vi "Create file path.vi"(11 "# photos":i32) -> (3 "Path OUT":path)   [LabVIEW 2018]
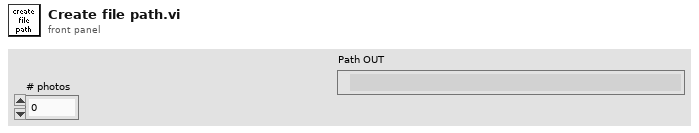
[diagram p1: front panel]
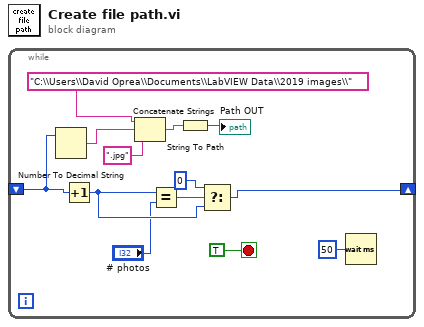
[diagram p0: block diagram]
diagram:
  n1 = while {
    shift-right: [w9] -> _
    shift-left: _ -> [w1]
    stop <- TRUE stop-if-true
    n2 = Number To Decimal String(number=w1) -> (decimal integer string=w8:string)  [unwired: 1 in]
    n3 = Increment(x=w1) -> (x+1=w10:i32)
    n4 = Concatenate Strings("C:\\Users\\David Oprea\\Documents\\LabVIEW Data\\2019 images\\", w8, ".jpg") -> (w6:string)
    n5 = Equal?(x=w10, y="# photos") -> (x = y?=w12:bool)
    n6 = String To Path(string=w6) -> (path=→"Path OUT":path)
    n7 = Select(t=0, s=w12, f=w10) -> (s? t:f=w9:i32)
    n8 = Wait (ms)(milliseconds to wait=u32 50) -> ()  [unwired: 1 out]
  }
